vi "Write Qsp.vi"(8 "error in (no error)":errorcluster, 10 "Qsp":dbl, 11 "Alicat Device in":refnum<class "Alicat Device.lvclass">) -> (0 "error out":errorcluster, 3 "Alicat Device out":refnum<class "Alicat Device.lvclass">)   [LabVIEW 2018, in "Alicat Lib.lvlib" / "Alicat Device.lvclass"]
uses:
  Alicat Device.lvclass
  Alicat Device.lvclass/Alicat Device.ctl
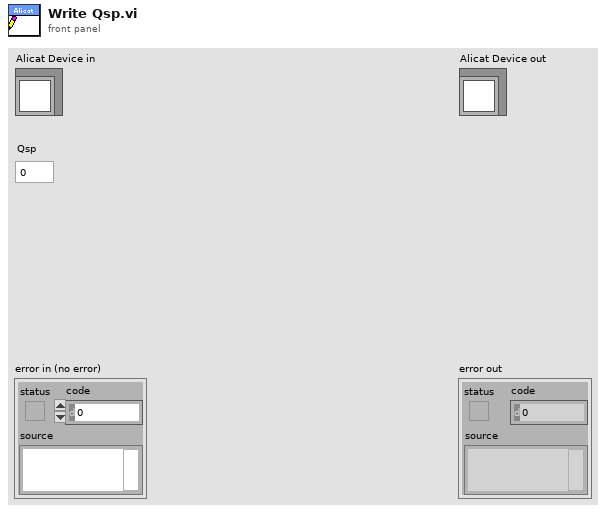
[diagram p1: front panel]
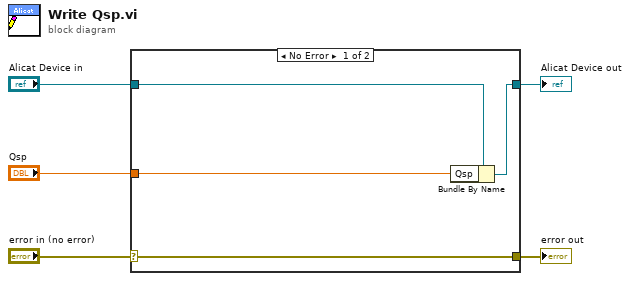
[diagram p0: block diagram]
diagram:
  n1 = case shown="No Error" "error in (no error)" {
    selector: "error in (no error)" -> [w9 w10]
    tunnel: [w9 w10] -> w4
    tunnel: [w7 w11] -> w2
    tunnel: "Alicat Device in" -> [w8 w11]
    tunnel: "Qsp" -> [w6 _]
    frame No Error {
      n2 = Bundle By Name(cluster=w8, "Qsp"=w6) -> (w7:refnum<class "Alicat Device.lvclass">)
    }
    frame Error {
    }
  }
  "error out" <- w4
  "Alicat Device out" <- w2
